vi "Close Connection.vi"(8 "error in (no error)":errorcluster, 11 "NXP in":refnum<class "NXP.lvclass">) -> (0 "error out":errorcluster, 3 "NXP out":refnum<class "NXP.lvclass">)   [LabVIEW 2020, in "NXP.lvclass"]
doc: "Método heredado del padre con un override"
uses:
  NXP.lvclass
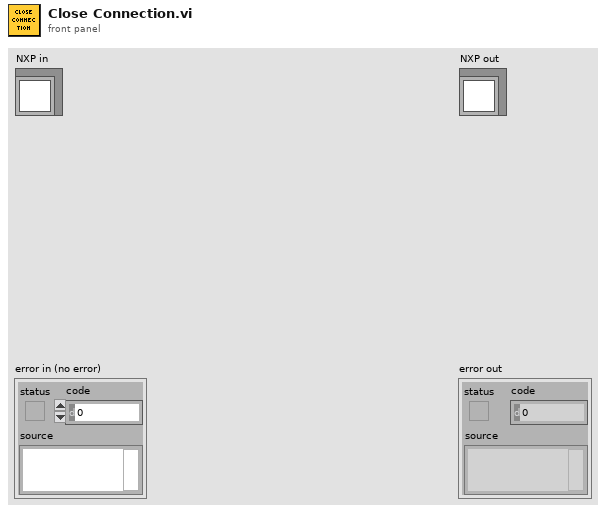
[diagram p1: front panel]
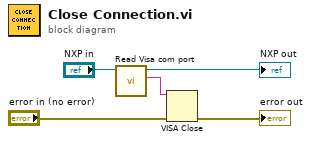
[diagram p0: block diagram]
diagram:
  n1 = call-dynamic "Read Visa com port.vi"("Serial device in"="NXP in") -> ("Visa com port"=w1:string, "Serial device out"=→"NXP out":refnum<class "NXP.lvclass">)  [unwired: 8 in, 1 out]
  n2 = VISA Close(VISA resource name=w1, error in (no error)="error in (no error)") -> (error out=→"error out":errorcluster)
